vi "NI-Digital Specific Logic.vi"(7 "pin map id":string, 8 "error in":errorcluster, 9 "channel list":string, 10 "Measurement Configuration":T2, 11 "instrument handle":refnum<k15>) -> (0 "error out":errorcluster, 2 "Measurement Results":T1, 3 "instrument handle out":refnum<k15>)   [LabVIEW 2020, in "NIDigitalSPI.lvlib"]
uses:
  NIDigitalSPI.lvlib
  Measurement Configuration.ctl
  Measurement Results.ctl
  <instrlib>/niDigital/niDigital.llb/niDigital Selected Function.ctl
  <instrlib>/niDigital/niDigital.llb/niDigital Load Specifications Levels and Timing (Single).vi
  <instrlib>/niDigital/niDigital.llb/niDigital Burst Pattern (Pass Fail).vi
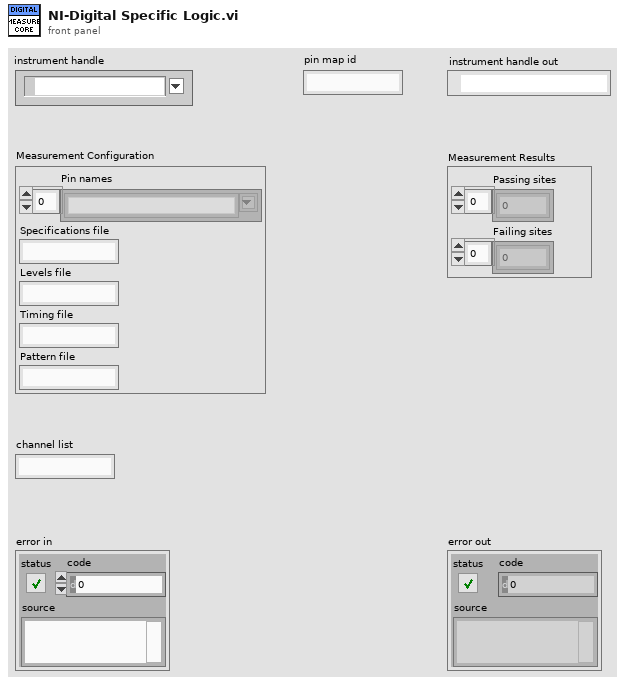
[diagram p1: front panel]
types:
  T1 = typedef "NIDigitalSPI.lvlib/Measurement Results.ctl" = cluster{"Passing sites":i32[], "Failing sites":i32[]}
  T2 = typedef "NIDigitalSPI.lvlib/Measurement Configuration.ctl" = cluster{"Pin names":string[], "Specifications file":string, "Levels file":string, "Timing file":string, "Pattern file":string}
  T3 = typedef "niDigital Selected Function.ctl" = i32
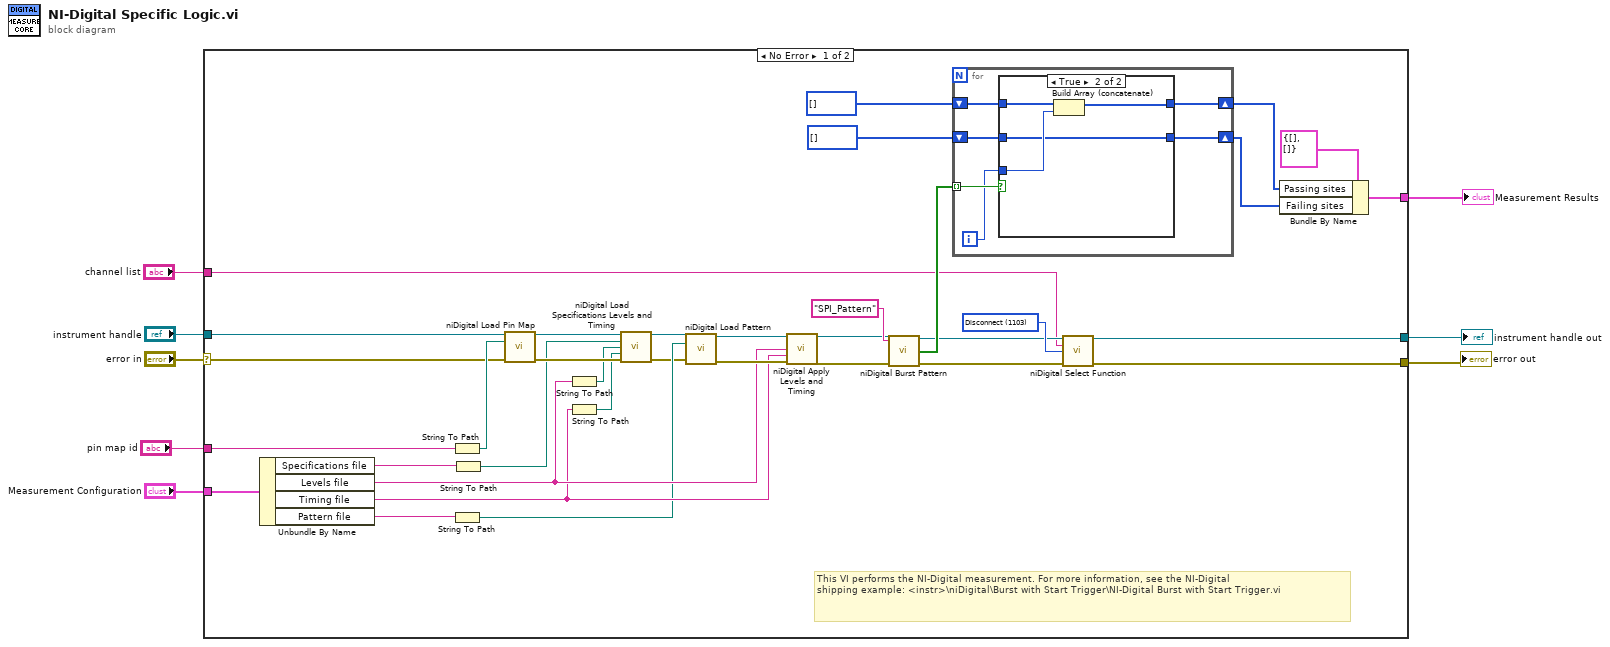
[diagram p0: block diagram]
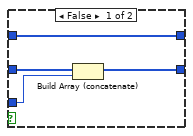
[diagram p2: hidden frame]
diagram:
  n1 = case shown="No Error" "error in" {
    selector: "error in" -> [w9 w58]
    tunnel: "Measurement Configuration" -> [w43 _]
    tunnel: [w41 _] -> w7
    tunnel: [w38 w58] -> w6
    tunnel: "instrument handle" -> [w40 w59]
    tunnel: [w39 w59] -> w4
    tunnel: "pin map id" -> [w24 _]
    tunnel: "channel list" -> [w19 _]
    frame No Error {
      w37 = T3 1103 items=["Digital"=1100, "PPMU"=1101, "Off"=1102, "Disconnect"=1103] ("function")
      # "This VI performs the NI-Digital measurement. For more information, see the NI-Digital\nshipping example: <instr>\\niDigital\\Burst with Start Trigger\\NI-Digital Burst with Start Trigger.vi"
      n2 = Unbundle By Name(w43) -> ("Specifications file"=w35:string, "Levels file"=w28:string, "Timing file"=w27:string, "Pattern file"=w36:string)
      n3 = String To Path(string=w24) -> (path=w15:path)
      n4 = String To Path(string=w36) -> (path=w16:path)
      n5 = String To Path(string=w35) -> (path=w14:path)
      n6 = call <instrlib>:"niDigital Load Pin Map.vi"("instrument handle"=w40, "pin map file"=w15, "error in"=w9) -> ("instrument handle out"=w17:refnum<k15>, "error out"=w18:errorcluster)  [unwired: 11 in]
      n7 = String To Path(string=w28) -> (path=w13:path)
      n8 = String To Path(string=w27) -> (path=w12:path)
      n9 = call-poly <instrlib>:"niDigital Load Specifications Levels and Timing.vi"("instrument handle"=w17, "specifications file path"=w14, "levels file path"=w13, "timing file path"=w12, "error in"=w18) -> ("instrument handle out"=w10:refnum<k15>, "error out"=w11:errorcluster)  [unwired: 9 in]
      n10 = call <instrlib>:"niDigital Load Pattern.vi"("instrument handle"=w10, "pattern file"=w16, "error in"=w11) -> ("instrument handle out"=w30:refnum<k15>, "error out"=w29:errorcluster)  [unwired: 11 in]
      n11 = call <instrlib>:"niDigital Apply Levels and Timing.vi"("instrument handle"=w30, "levels sheet"=w28, "timing sheet"=w27, "error in"=w29) -> ("instrument handle out"=w25:refnum<k15>, "error out"=w26:errorcluster)  [unwired: 10 in]
      n12 = call-poly <instrlib>:"niDigital Burst Pattern.vi"("instrument handle"=w25, "start label"="SPI_Pattern", "error in"=w26) -> ("instrument handle out"=w33:refnum<k15>, "pass"=w34:bool[], "error out"=w32:errorcluster)  [unwired: 10 in]
      n13 = for {
        tunnel: w34 -> [w49] mode=indexing
        shift-right: [w48] -> w21
        shift-left: i32[] [] -> [w47]
        shift-right: [w45] -> w20
        shift-left: i32[] [] -> [w46]
        i -> [w44]
        n14 = case shown="True" w49 {
          tunnel: w44 -> [w51 w56]
          tunnel: [w53 w57] -> w48
          tunnel: w47 -> [w53 w55]
          tunnel: w46 -> [w52 w54]
          tunnel: [w50 w54] -> w45
          frame False {
            n15 = Build Array (concatenate)(w52, w51) -> (w50:i32[])
          }
          frame True {
            n16 = Build Array (concatenate)(w55, w56) -> (w57:i32[])
          }
        }
      }
      n17 = call <instrlib>:"niDigital Select Function.vi"("instrument handle"=w33, "channel list"=w19, "function"=w37, "error in"=w32) -> ("instrument handle out"=w39:refnum<k15>, "error out"=w38:errorcluster)  [unwired: 10 in]
      n18 = Bundle By Name(cluster=T1 {"Passing sites"=[], "Failing sites"=[]} ("Measurement Results"), "Passing sites"=w21, "Failing sites"=w20) -> (w41:T1)
    }
    frame Error {
    }
  }
  "Measurement Results" <- w7
  "error out" <- w6
  "instrument handle out" <- w4
